vi "buttons pressed.vi"(11 "NXT 2":T1 {"Connection" items=["USB", "Bluetooth", "USB then Bluetooth", "Last Connection", "Preference"]}) -> (1 "Buttons pressed":T2 items=["None", "Center", "Left", "C+L", "Right", "C+R", "C+L", "All"], 3 "NXT":T1 {"Connection" items=["USB", "Bluetooth", "USB then Bluetooth", "Last Connection", "Preference"]})   [LabVIEW 2009]
doc: "Button Pressed Values:\n0 - None\n1 - Center\n2 - Left\n3 - Center + Left\n4 - Right\n5 - Center + Right\n6 - Left + Right\n7 - All"
uses:
  <vilib>/NXT/Subs/LVHSConnector.ctl
  buttons pressed.ctl
  <vilib>/NXT/Block Support/NXT_ButtonSelector.ctl
  <vilib>/NXT/Dual Mode Library/Sensors/readNXTButton.vi
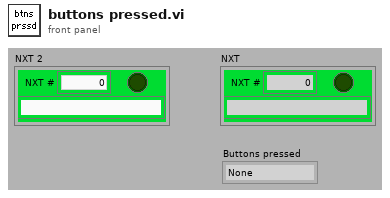
[diagram p1: front panel]
types:
  T1 = typedef "LVHSConnector.ctl" = cluster{"error":errorcluster, "address":string, "NXT #":i32, "Show Error":bool, "Connection":u16}
  T2 = typedef "buttons pressed.ctl" = u8
  T3 = typedef "NXT_ButtonSelector.ctl" = u16
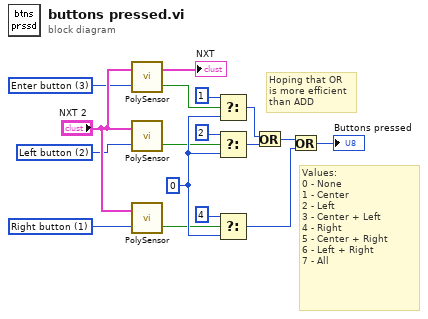
[diagram p0: block diagram]
diagram:
  w7 = u8 0
  w6 = T3 1 items=["Enter button"=3, "Left button"=2, "Right button"=1] ("Button (Enter button)")
  w5 = T3 2 items=["Enter button"=3, "Left button"=2, "Right button"=1] ("Button (Enter button)")
  w4 = T3 3 items=["Enter button"=3, "Left button"=2, "Right button"=1] ("Button (Enter button)")
  # "Values:\n0 - None\n1 - Center\n2 - Left\n3 - Center + Left\n4 - Right\n5 - Center + Right\n6 - Left + Right\n7 - All"
  # "Hoping that OR\nis more efficient\nthan ADD"
  n1 = call-poly <vilib>:"PolySensor.vi"("Button (Enter button)"=w4, "NXT"="NXT 2") -> ("Yes/No"=w3:bool, "NXT"=→"NXT":T1)  [unwired: 1 in]
  n2 = call-poly <vilib>:"PolySensor.vi"("Button (Enter button)"=w5, "NXT"="NXT 2") -> ("Yes/No"=w2:bool)  [unwired: 1 in, 1 out]
  n3 = call-poly <vilib>:"PolySensor.vi"("Button (Enter button)"=w6, "NXT"="NXT 2") -> ("Yes/No"=w1:bool)  [unwired: 1 in, 1 out]
  n4 = Select(t=u8 1, s=w3, f=w7) -> (s? t:f=w12:u8)
  n5 = Select(t=u8 2, s=w2, f=w7) -> (s? t:f=w13:u8)
  n6 = Select(t=u8 4, s=w1, f=w7) -> (s? t:f=w14:u8)
  n7 = Or(x=w12, y=w13) -> (x .or. y?=w15:u8)
  n8 = Or(x=w15, y=w14) -> (x .or. y?=→"Buttons pressed":u8)
